vi "convert_json_string_to_ui_element.vi"(0 "json string":string, 11 "error in (no error)":errorcluster) -> (4 "labview structure":T4, 15 "error out":errorcluster)   [LabVIEW 2020]
uses:
  <vilib>/Utility/miscctls.llb/LVBoundsTypeDef.ctl
  <vilib>/Utility/miscctls.llb/LVPositionTypeDef.ctl
  <vilib>/Utility/miscctls.llb/LVPointTypeDef.ctl
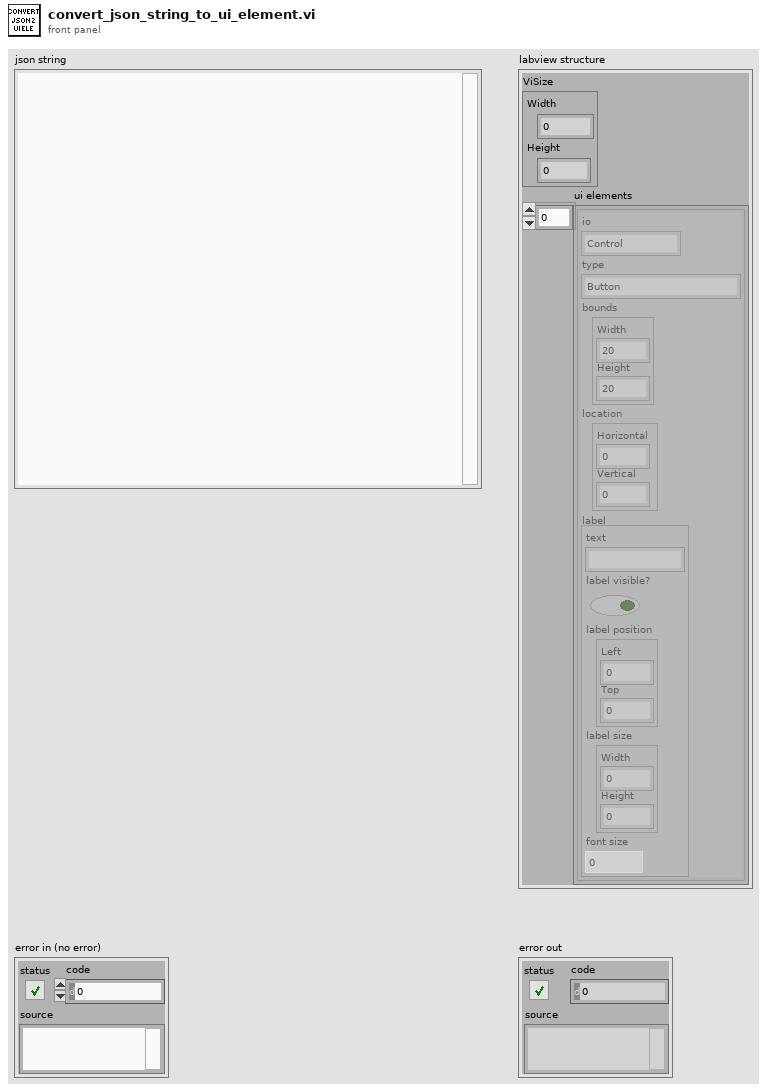
[diagram p1: front panel]
types:
  T1 = typedef "LVBoundsTypeDef.ctl" = cluster{"Width":u32, "Height":u32}
  T2 = typedef "LVPointTypeDef.ctl" = cluster{"Horizontal":i16, "Vertical":i16}
  T3 = typedef "LVPositionTypeDef.ctl" = cluster{"Left":i32, "Top":i32}
  T4 = cluster{"ViSize":cluster{"Width":i16, "Height":i16}, "ui elements":cluster{"io":string, "type":string, "bounds":T1, "location":T2, "label":cluster{"text":string, "label visible?":bool, "label position":T3, "label size":T1, "font size":u32}}[]}
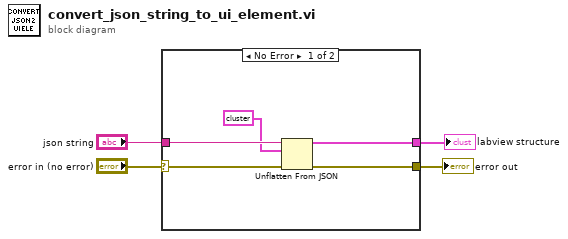
[diagram p0: block diagram]
diagram:
  n1 = case shown="No Error" "error in (no error)" {
    selector: "error in (no error)" -> [w6 w10]
    tunnel: [w7 w10] -> w3
    tunnel: [w9 _] -> w1
    tunnel: "json string" -> [w8 _]
    frame No Error {
      n2 = Unflatten From JSON(JSON string=w8, type and defaults=T4 {"ViSize"={"Width"=300, "Height"=250}, "ui elements"=[{"io"="Control", "type"="String Control (system)", "bounds"={"Width"=200, "Height"=25}, "location"={"Horizontal"=70, "Vertical"=10}, "label"={"text"="Email", "label visible?"=TRUE, "label position"={"Left"=10, "Top"=15}, "label size"={"Width"=50, "Height"=15}, "font size"=0}}, {"io"="Control", "type"="String Control (system)", "bounds"={"Width"=200, "Height"=25}, "location"={"Horizontal"=70, "Vertical"=45}, "label"={"text"="Name", "label visible?"=TRUE, "label position"={"Left"=10, "Top"=50}, "label size"={"Width"=50, "Height"=15}, "font size"=0}}, {"io"="Control", "type"="String Control (system)", "bounds"={"Width"=200, "Height"=25}, "location"={"Horizontal"=70, "Vertical"=80}, "label"={"text"="State", "label visible?"=TRUE, "label position"={"Left"=10, "Top"=85}, "label size"={"Width"=50, "Height"=15}, "font size"=0}}, {"io"="Control", "type"="Combo Box (modern)", "bounds"={"Width"=200, "Height"=25}, "location"={"Horizontal"=70, "Vertical"=115}, "label"={"text"="Country", "label visible?"=TRUE, "label position"={"Left"=10, "Top"=120}, "label size"={"Width"=60, "Height"=15}, "font size"=0}}, {"io"="Control", "type"="String Control (system)", "bounds"={"Width"=120, "Height"=25}, "location"={"Horizontal"=110, "Vertical"=150}, "label"={"text"="Begun studies", "label visible?"=TRUE, "label position"={"Left"=10, "Top"=155}, "label size"={"Width"=90, "Height"=15}, "font size"=0}}, {"io"="Control", "type"="Push Button", "bounds"={"Width"=25, "Height"=25}, "location"={"Horizontal"=235, "Vertical"=150}, "label"={"text"="Calendar Button", "label visible?"=FALSE, "label position"={"Left"=235, "Top"=150}, "label size"={"Width"=0, "Height"=0}, "font size"=0}}, {"io"="Control", "type"="String Control (system)", "bounds"={"Width"=200, "Height"=25}, "location"={"Horizontal"=70, "Vertical"=185}, "label"={"text"="Notes", "label visible?"=TRUE, "label position"={"Left"=10, "Top"=190}, "label size"={"Width"=50, "Height"=15}, "font size"=0}}]} ("labview structure"), error in (no error)=w6) -> (value=w9:T4, error out=w7:errorcluster)  [unwired: 4 in]
    }
    frame Error {
    }
  }
  "error out" <- w3
  "labview structure" <- w1
